vi "Set VolatusAPI.vi"(10 "VolatusAPI":refnum<class "VolatusAPI.lvclass">, 11 "Module in":refnum<class "Module.lvclass">) -> (3 "Module out":refnum<class "Module.lvclass">)   [LabVIEW 2020, in "Volatus.lvlib" / "Module.lvclass"]
uses:
  Module.lvclass
  VolatusAPI/VolatusAPI.lvclass
  Module.lvclass/Module.ctl
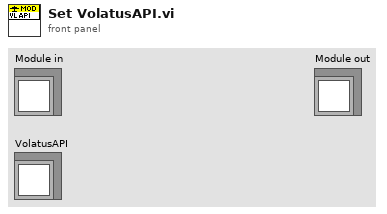
[diagram p1: front panel]
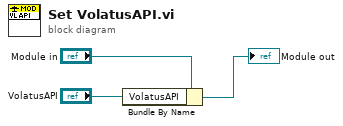
[diagram p0: block diagram]
diagram:
  n1 = Bundle By Name(cluster="Module in", "VolatusAPI"="VolatusAPI") -> (→"Module out":refnum<class "Module.lvclass">)
